vi "OAT Segment Averaging.vi"(6 "boundaries":i32[](array[numeric]), 7 "Y [EU]":dbl[](array[numeric]) format="%.2f") -> (3 "energy level in ranges [EU^2]":dbl[](array[numeric]) format="%.2f")   [LabVIEW 2017, in "SoundVib_Gabor.lvlib"]
uses:
  <vilib>/addons/Sound and Vibration/Order Analysis/Gabor Order Tracking/SoundVib_Gabor.lvlib
  <vilib>/Analysis/baseanly.llb/Mean (DBL).vi
  <vilib>/Analysis/NI_AALBase.lvlib
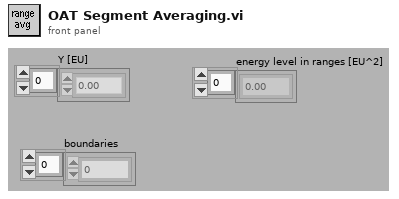
[diagram p1: front panel]
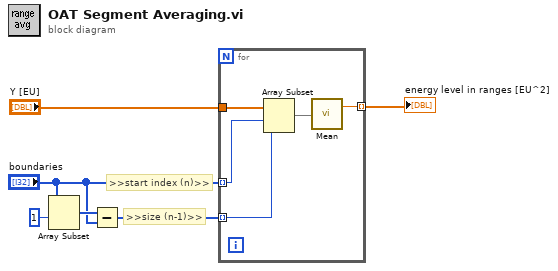
[diagram p0: block diagram]
diagram:
  # ">>size (n-1)>>"
  # ">>start index (n)>>"
  n1 = Array Subset(array="boundaries", index=1 ("Array Index")) -> (w3:i32[])  [unwired: 1 in]
  n2 = Subtract(x=w3, y="boundaries") -> (x-y=w1:i32[])
  n3 = for {
    tunnel: "Y [EU]" -> [w11]
    tunnel: [w7] -> w5 mode=indexing
    tunnel: "boundaries" -> [w10] mode=indexing
    tunnel: w1 -> [w9] mode=indexing
    n4 = Array Subset(array=w11, index=w10, length=w9) -> (w8:dbl[])
    n5 = call-poly <vilib>:"Mean.vi"("X"=w8) -> ("mean"=w7:dbl)  [unwired: 1 out]
  }
  "energy level in ranges [EU^2]" <- w5
